vi "SessionManagementService GetMultiplexerSessions.vi"(6 "contextId":T1, 8 "error in":errorcluster, 9 "timeout (ms)":i32=-1, 10 "Request Data":T6, 11 "gRPC ID":T1) -> (0 "error out":errorcluster, 2 "Response Data":T2, 3 "gRPC ID out":T1)   [LabVIEW 2021, in "ni.measurementlink.sessionmanagement.v1.api.lvlib"]
uses:
  ni.measurementlink.sessionmanagement.v1.api.lvlib
  <vilib>/gRPC/LabVIEW gRPC Library/Shared/grpcId.ctl
  RPC Messages/ni_measurementlink_sessionmanagement_v1_GetMultiplexerSessionsRequest.ctl
  RPC Messages/ni_measurementlink_PinMapContext.ctl
  RPC Messages/ni_measurementlink_sessionmanagement_v1_GetMultiplexerSessionsResponse.ctl
  RPC Messages/ni_measurementlink_sessionmanagement_v1_MultiplexerSessionInformation.ctl
  RPC Messages/nidevice_grpc_Session.ctl
  RPC Messages/ni_measurementlink_sessionmanagement_v1_MultiplexerSessionInformation_AnnotationsEntry.ctl
  RPC Messages/ni_measurementlink_sessionmanagement_v1_GetMultiplexerSessionsResponse_Flat.ctl
  RPC Messages/ni_measurementlink_sessionmanagement_v1_MultiplexerSessionInformation_Flat.ctl
  RPC Messages/nidevice_grpc_Session_Flat.ctl
  RPC Messages/ni_measurementlink_sessionmanagement_v1_MultiplexerSessionInformation_AnnotationsEntry_Flat.ctl
  14035477-4c25-4107-8ed5-d0c4ef420ce5.vi
  RPC Messages/RichToFlatni_measurementlink_PinMapContext.vi
  <vilib>/gRPC/LabVIEW gRPC Library/Shared/TranslateGrpcError.vi
  <vilib>/gRPC/LabVIEW gRPC Library/Shared/Wait On Occurrence.vi
  RPC Messages/FlatToRichni_measurementlink_sessionmanagement_v1_MultiplexerSessionInformation.vi
  <vilib>/gRPC/LabVIEW gRPC Library/Shared/Is Feature Enabled.vi
  RPC Messages/FlatToRichnidevice_grpc_Session.vi
  RPC Messages/FlatToRichni_measurementlink_sessionmanagement_v1_MultiplexerSessionInformation_AnnotationsEntry.vi
  <vilib>/gRPC/LabVIEW gRPC Library/Server API/Server/Get Server DLL Path.vi
  <vilib>/Utility/error.llb/Error Cluster From Error Code.vi
  <vilib>/gRPC/LabVIEW gRPC Library/grpc-lvsupport-release.lvlib
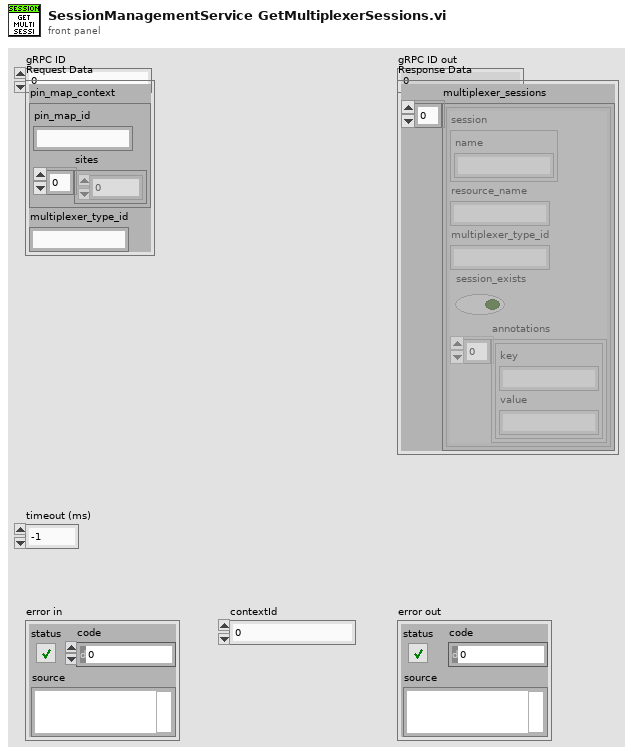
[diagram p1: front panel]
types:
  T1 = typedef "grpc-lvsupport-release.lvlib/grpcId.ctl" = u64
  T2 = typedef "ni.measurementlink.sessionmanagement.v1.api.lvlib/ni_measurementlink_sessionmanagement_v1_GetMultiplexerSessionsResponse.ctl" = cluster{"multiplexer_sessions":T3[]}
  T3 = typedef "ni.measurementlink.sessionmanagement.v1.api.lvlib/ni_measurementlink_sessionmanagement_v1_MultiplexerSessionInformation.ctl" = cluster{"session":T4, "resource_name":string, "multiplexer_type_id":string, "session_exists":bool, "annotations":T5[]}
  T4 = typedef "ni.measurementlink.sessionmanagement.v1.api.lvlib/nidevice_grpc_Session.ctl" = cluster{"name":string}
  T5 = typedef "ni.measurementlink.sessionmanagement.v1.api.lvlib/ni_measurementlink_sessionmanagement_v1_MultiplexerSessionInformation_AnnotationsEntry.ctl" = cluster{"key":string, "value":string}
  T6 = typedef "ni.measurementlink.sessionmanagement.v1.api.lvlib/ni_measurementlink_sessionmanagement_v1_GetMultiplexerSessionsRequest.ctl" = cluster{"pin_map_context":T7, "multiplexer_type_id":string}
  T7 = typedef "ni.measurementlink.sessionmanagement.v1.api.lvlib/ni_measurementlink_PinMapContext.ctl" = cluster{"pin_map_id":string, "sites":i32[]}
  T8 = typedef "ni.measurementlink.sessionmanagement.v1.api.lvlib/ni_measurementlink_sessionmanagement_v1_GetMultiplexerSessionsResponse_Flat.ctl" = cluster{"multiplexer_sessions":T9[]}
  T9 = typedef "ni.measurementlink.sessionmanagement.v1.api.lvlib/ni_measurementlink_sessionmanagement_v1_MultiplexerSessionInformation_Flat.ctl" = cluster{"session":T10, "resource_name":string, "multiplexer_type_id":string, "session_exists":bool, "annotations":T11[]}
  T10 = typedef "ni.measurementlink.sessionmanagement.v1.api.lvlib/nidevice_grpc_Session_Flat.ctl" = cluster{"name":string}
  T11 = typedef "ni.measurementlink.sessionmanagement.v1.api.lvlib/ni_measurementlink_sessionmanagement_v1_MultiplexerSessionInformation_AnnotationsEntry_Flat.ctl" = cluster{"key":string, "value":string}
  T12 = typedef "ni.measurementlink.sessionmanagement.v1.api.lvlib/ni_measurementlink_sessionmanagement_v1_GetMultiplexerSessionsRequest_Flat.ctl" = cluster{"pin_map_context":T13, "multiplexer_type_id":string}
  T13 = typedef "ni.measurementlink.sessionmanagement.v1.api.lvlib/ni_measurementlink_PinMapContext_Flat.ctl" = cluster{"pin_map_id":string, "sites":i32[]}
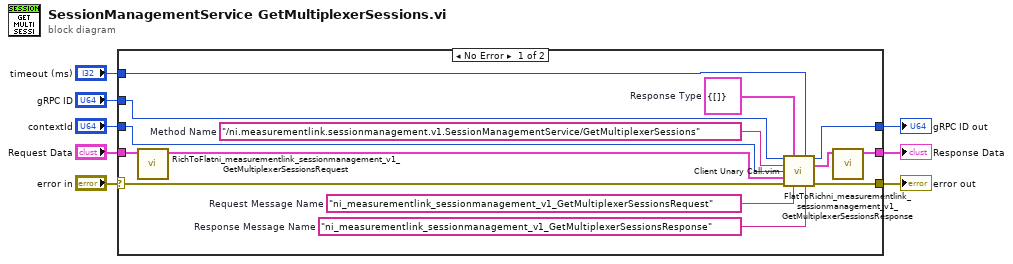
[diagram p0: block diagram]
diagram:
  n1 = case shown="No Error" "error in" {
    selector: "error in" -> [w18 w23]
    tunnel: [w17 w23] -> w7
    tunnel: "gRPC ID" -> [w16 w24]
    tunnel: [w15 w24] -> w5
    tunnel: "Request Data" -> [w12 _]
    tunnel: [w9 _] -> w3
    tunnel: "timeout (ms)" -> [w14 _]
    tunnel: "contextId" -> [w13 _]
    frame No Error {
      w19 = "ni_measurementlink_sessionmanagement_v1_GetMultiplexerSessionsResponse"  # Response Message Name
      w20 = "ni_measurementlink_sessionmanagement_v1_GetMultiplexerSessionsRequest"  # Request Message Name
      w21 = T8 {"multiplexer_sessions"=[]}  # Response Type
      w22 = "/ni.measurementlink.sessionmanagement.v1.SessionManagementService/GetMultiplexerSessions"  # Method Name
      n2 = call "RichToFlatni_measurementlink_sessionmanagement_v1_GetMultiplexerSessionsRequest.vi"("InputCluster"=w12) -> ("OutputCluster"=w11:T12)  [unwired: 10 in]
      n3 = call "Client Unary Call.vim"("ClientID in"=w16, "Response Type"=w21, "timeout (ms)"=w14, "Method Name"=w22, "contextId"=w13, "Request Data"=w11, "error in"=w18, "Request Message Name"=w20, "Response Message Name"=w19) -> ("ClientID out"=w15:u64, "Response Data"=w10:T8, "error out"=w17:errorcluster)  [unwired: 4 in]
      n4 = call "FlatToRichni_measurementlink_sessionmanagement_v1_GetMultiplexerSessionsResponse.vi"("InputCluster"=w10) -> ("OutputCluster"=w9:T2)  [unwired: 10 in]
    }
    frame Error {
    }
  }
  "error out" <- w7
  "gRPC ID out" <- w5
  "Response Data" <- w3
